vi "Read Battery Voltage.vi"() -> (2 "Voltage":dbl)   [LabVIEW 2013]
uses:
  <vilib>/Rock Robotics/WPI/AnalogModule/WPI_AnalogModuleDevStatus.ctl
  <vilib>/Rock Robotics/SystemInterfaces/Typedef/FPGA_TypedefAnalogModule.ctl
  <vilib>/Rock Robotics/SystemInterfaces/AI/FPGA_AIChannel.ctl
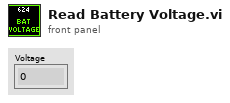
[diagram p1: front panel]
types:
  T1 = typedef "FPGA_AIChannel.ctl" = enum8{"AI 1", "AI 2", "AI 3", "AI 4", "AI 5", "AI 6", "AI 7", "AI 8", "Invalid"}
  T2 = typedef "WPI_AnalogModuleDevStatus.ctl" = cluster{"DevStatus":errorcluster, "Analog Module":T3}
  T3 = typedef "FPGA_TypedefAnalogModule.ctl" = enum16{"Analog Module 1", "Analog Module 2"}
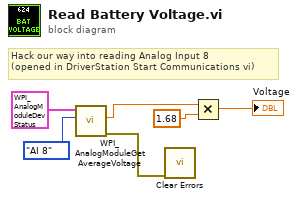
[diagram p0: block diagram]
diagram:
  # "Hack our way into reading Analog Input 8\n(opened in DriverStation Start Communications vi)"
  n1 = call <vilib>:"WPI_AnalogModuleGetAverageVoltage.vi"("Channel"=FPGA_AIChannel."AI 8", "AnalogModuleDevStatus"=T2 {"DevStatus"={"status"=FALSE, "code"=0, "source"=""}, "Analog Module"=enum."Analog Module 1"}) -> ("error out"=w2:errorcluster, "Average Voltage"=w1:dbl)  [unwired: 1 in, 7 out]
  n2 = call <vilib>:"Clear Errors.vi"("error in (no error)"=w2) -> ()  [unwired: 6 in, 1 out]
  n3 = Multiply(x=w1, y=1.68 ("x")) -> (x*y=→"Voltage":dbl)
